vi "DAQmx Initialise.vi"(8 "error in":errorcluster) -> (0 "error out":errorcluster, 3 "task out":refnum<k21>)   [LabVIEW 2018]
uses:
  <vilib>/DAQmx/create/channels.llb/DAQmx Create Channel (AI-Voltage-Basic).vi
  <vilib>/DAQmx/create/channels.llb/DAQmx Create Channel (TEDS-AI-Voltage-Basic).vi
  <vilib>/DAQmx/configure/timing.llb/DAQmx Timing (Sample Clock).vi
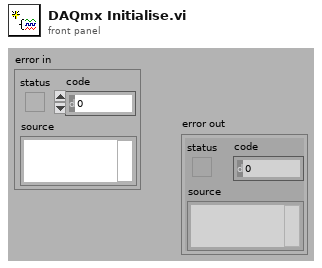
[diagram p1: front panel]
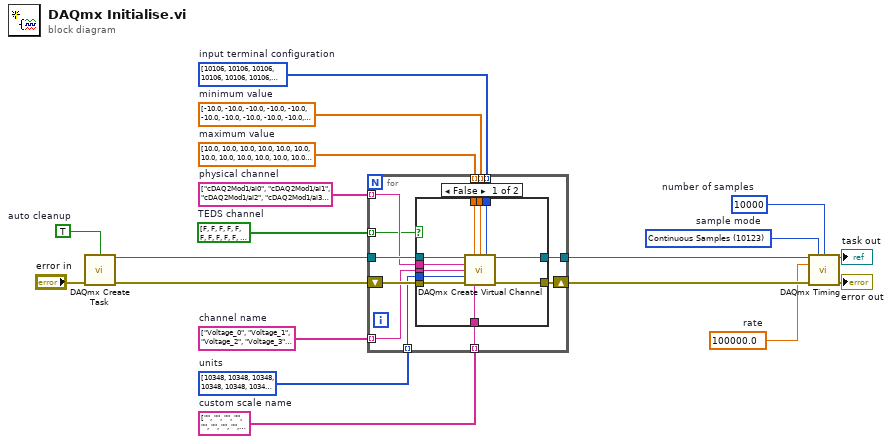
[diagram p0: block diagram]
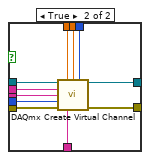
[diagram p2: hidden frame]
diagram:
  w1 = 10123 items=["Finite Samples"=10178, "Continuous Samples"=10123, "Hardware Timed Single Point"=12522]  # sample mode
  w2 = 10000  # number of samples
  w3 = 100000.0  # rate
  w7 = bool[] [FALSE, FALSE, FALSE, FALSE, FALSE, FALSE, FALSE, FALSE, FALSE, FALSE, FALSE, FALSE, FALSE, FALSE, FALSE, FALSE, FALSE, FALSE, FALSE, FALSE, FALSE, FALSE, FALSE, FALSE, FALSE, FALSE, FALSE, FALSE]  # TEDS channel
  w12 = string[] ["", "", "", "", "", "", "", "", "", "", "", "", "", "", "", "", "", "", "", "", "", "", "", "", "", "", "", ""]  # custom scale name
  w11 = i32[] [10348, 10348, 10348, 10348, 10348, 10348, 10348, 10348, 10348, 10348, 10348, 10348, 10348, 10348, 10348, 10348, 10348, 10348, 10348, 10348, 10348, 10348, 10348, 10348, 10348, 10348, 10348, 10348] items=["Volts"=10348, "From TEDS"=12516, "From Custom Scale"=10065]  # units
  w10 = string[] ["Voltage_0", "Voltage_1", "Voltage_2", "Voltage_3", "Voltage_4", "Voltage_5", "Voltage_6", "Voltage_7", "Voltage_8", "Voltage_9", "Voltage_10", "Voltage_11", "Voltage_12", "Voltage_13", "Voltage_14", "Voltage_15", "Voltage_16", "Voltage_17", "Voltage_18", "Voltage_19", "Voltage_20", "Voltage_21", "Voltage_22", "Voltage_23", "Voltage_24", "Voltage_25", "Voltage_26", "Voltage_27"]  # channel name
  w9 = string[] ["cDAQ2Mod1/ai0", "cDAQ2Mod1/ai1", "cDAQ2Mod1/ai2", "cDAQ2Mod1/ai3", "cDAQ2Mod2/ai0", "cDAQ2Mod2/ai1", "cDAQ2Mod2/ai2", "cDAQ2Mod2/ai3", "cDAQ2Mod3/ai0", "cDAQ2Mod3/ai1", "cDAQ2Mod3/ai2", "cDAQ2Mod3/ai3", "cDAQ2Mod4/ai0", "cDAQ2Mod4/ai1", "cDAQ2Mod4/ai2", "cDAQ2Mod4/ai3", "cDAQ2Mod5/ai0", "cDAQ2Mod5/ai1", "cDAQ2Mod5/ai2", "cDAQ2Mod5/ai3", "cDAQ2Mod6/ai0", "cDAQ2Mod6/ai1", "cDAQ2Mod6/ai2", "cDAQ2Mod6/ai3", "cDAQ2Mod7/ai0", "cDAQ2Mod7/ai1", "cDAQ2Mod7/ai2", "cDAQ2Mod7/ai3"]  # physical channel
  w13 = dbl[] [10.0, 10.0, 10.0, 10.0, 10.0, 10.0, 10.0, 10.0, 10.0, 10.0, 10.0, 10.0, 10.0, 10.0, 10.0, 10.0, 10.0, 10.0, 10.0, 10.0, 10.0, 10.0, 10.0, 10.0, 10.0, 10.0, 10.0, 10.0]  # maximum value
  w14 = dbl[] [-10.0, -10.0, -10.0, -10.0, -10.0, -10.0, -10.0, -10.0, -10.0, -10.0, -10.0, -10.0, -10.0, -10.0, -10.0, -10.0, -10.0, -10.0, -10.0, -10.0, -10.0, -10.0, -10.0, -10.0, -10.0, -10.0, -10.0, -10.0]  # minimum value
  w15 = i32[] [10106, 10106, 10106, 10106, 10106, 10106, 10106, 10106, 10106, 10106, 10106, 10106, 10106, 10106, 10106, 10106, 10106, 10106, 10106, 10106, 10106, 10106, 10106, 10106, 10106, 10106, 10106, 10106] items=["default"=-1, "RSE"=10083, "NRSE"=10078, "Differential"=10106, "Pseudodifferential"=12529]  # input terminal configuration
  w17 = TRUE  # auto cleanup
  n1 = call <vilib>:"DAQmx Create Task.vi"("auto cleanup"=w17, "error in"="error in") -> ("task out"=w16:refnum<k21>, "error out"=w18:errorcluster)  [unwired: 12 in]
  n2 = for {
    tunnel: w16 -> [w28]
    tunnel: w15 -> [w29] mode=indexing
    tunnel: w14 -> [w30] mode=indexing
    tunnel: w13 -> [w31] mode=indexing
    tunnel: w12 -> [w21] mode=indexing
    tunnel: w11 -> [w22] mode=indexing
    tunnel: w10 -> [w24] mode=indexing
    tunnel: w9 -> [w23] mode=indexing
    tunnel: [w26] -> w4
    shift-right: [w25] -> w8
    shift-left: w18 -> [w27]
    tunnel: w7 -> [w20] mode=indexing
    n3 = case shown="False" w20 {
      tunnel: w31 -> [w42 w47]
      tunnel: w30 -> [w41 w48]
      tunnel: w29 -> [w40 w49]
      tunnel: w28 -> [w39 w53]
      tunnel: w27 -> [w38 w52]
      tunnel: [w37 w50] -> w26
      tunnel: [w36 w51] -> w25
      tunnel: w24 -> [w35 w45]
      tunnel: w23 -> [w34 w46]
      tunnel: w22 -> [w33 w44]
      tunnel: w21 -> [w32 w43]
      frame False {
        n4 = call-poly <vilib>:"DAQmx Create Virtual Channel.vi"("task in"=w39, "maximum value"=w42, "minimum value"=w41, "input terminal configuration"=w40, "physical channels"=w34, "name to assign"=w35, "units"=w33, "error in"=w38, "custom scale name"=w32) -> ("task out"=w37:refnum<k21>, "error out"=w36:errorcluster)  [unwired: 5 in]
      }
      frame True {
        n5 = call-poly <vilib>:"DAQmx Create Virtual Channel.vi"("task in"=w53, "maximum value"=w47, "minimum value"=w48, "input terminal configuration"=w49, "physical channels"=w46, "name to assign"=w45, "units"=w44, "error in"=w52, "custom scale name"=w43) -> ("task out"=w50:refnum<k21>, "error out"=w51:errorcluster)  [unwired: 5 in]
      }
    }
  }
  n6 = call-poly <vilib>:"DAQmx Timing.vi"("task/channels in"=w4, "sample mode"=w1, "samples per channel"=w2, "rate"=w3, "error in"=w8) -> ("task out"=→"task out":refnum<k21>, "error out"=→"error out":errorcluster)  [unwired: 9 in]
